vi "ControlStreamWindow.vi"(0 "reference in":refnum<class "Streamer.lvclass">, 2 "ShowProcessWindow":bool, 5 "Error In":errorcluster) -> (14 "reference out":refnum<class "Streamer.lvclass">, 19 "Error Out":errorcluster)   [LabVIEW 2023, in "Streamer.lvclass"]
uses:
  Streamer.lvclass
  Streamer.lvclass/Streamer.ctl
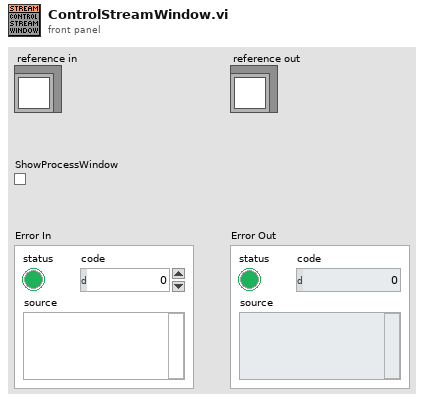
[diagram p1: front panel]
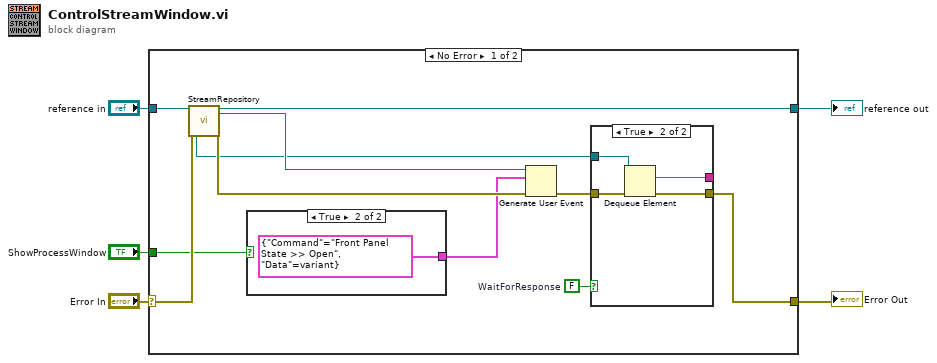
[diagram p0: block diagram]
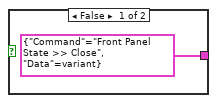
[diagram p2: hidden frame]
diagram:
  n1 = case shown="No Error" "Error In" {
    selector: "Error In" -> [w16 w25]
    tunnel: [w9 w25] -> w4
    tunnel: [w14 w24] -> w2
    tunnel: "reference in" -> [w15 w24]
    tunnel: "ShowProcessWindow" -> [w7 _]
    frame No Error {
      w12 = FALSE  # WaitForResponse
      n2 = call "StreamRepository.vi"("reference in"=w15, "Error In"=w16) -> ("QueueFromProcess"=w8:refnum<queue>, "reference out"=w14:refnum<class "Streamer.lvclass">, "EventsToProcess"=w13:refnum<user-event>, "Error Out"=w10:errorcluster)  [unwired: 10 in, 4 out]
      n3 = case shown="True" w7 {
        tunnel: [cluster{"Command":string, "Data":variant} {"Command"="Front Panel State >> Close", "Data"=variant} ("MessageToProcess") cluster{"Command":string, "Data":variant} {"Command"="Front Panel State >> Open", "Data"=variant} ("MessageToProcess")] -> w6
        frame False {
        }
        frame True {
        }
      }
      n4 = Generate User Event(user event=w13, event data cluster=w6, error in=w10) -> (error out=w11:errorcluster)  [unwired: 1 in, 1 out]
      n5 = case shown="True" w12 {
        tunnel: w11 -> [w19 w23]
        tunnel: [_ w22] -> _
        tunnel: [w19 w21] -> w9
        tunnel: w8 -> [_ w20]
        frame False {
        }
        frame True {
          n6 = Dequeue Element(queue=w20, error in (no error)=w23) -> (element=w22:string, error out=w21:errorcluster)  [unwired: 1 in, 2 out]
        }
      }
    }
    frame Error {
    }
  }
  "Error Out" <- w4
  "reference out" <- w2
